vi "Moving Average (multiple).vi"(6 "Window Unit (points)":enum16{"Points", "Data"}(ring), 8 "error in (no error)":errorcluster, 10 "Window":dbl, 11 "XY-data":cluster{"X-array":dbl[], "Y-array":dbl[]}[](array[cluster])) -> (0 "error out":errorcluster, 3 "XY-data out":cluster{"X-array":dbl[], "Y-array":dbl[]}[](array[cluster]) {"Y-array" format="%.2p"; "X-array" format="%.2p"})   [LabVIEW 2019, in "xy_utilities.lvlib"]
doc: "Apply a moving average <b>XY-data</b>'s Y-Array according to <b>window</b>\n\nWire data to the data input to determine the polymorphic instance to use or manually select the instance."
uses:
  xy_utilities.lvlib
  Private/X Units.vi
  Private/X Array Range to Index.vi
  <vilib>/Analysis/3filter.llb/Smoothing Filter Coefficients.vi
  <vilib>/Analysis/3filter.llb/IIR Filter.vi
  <vilib>/Analysis/3filter.llb/IIR Filter (DBL).vi
  <vilib>/Utility/error.llb/Error Cluster From Error Code.vi
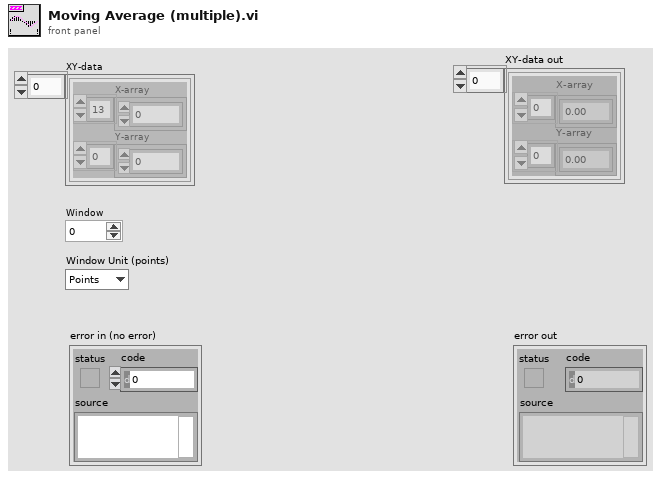
[diagram p1: front panel]
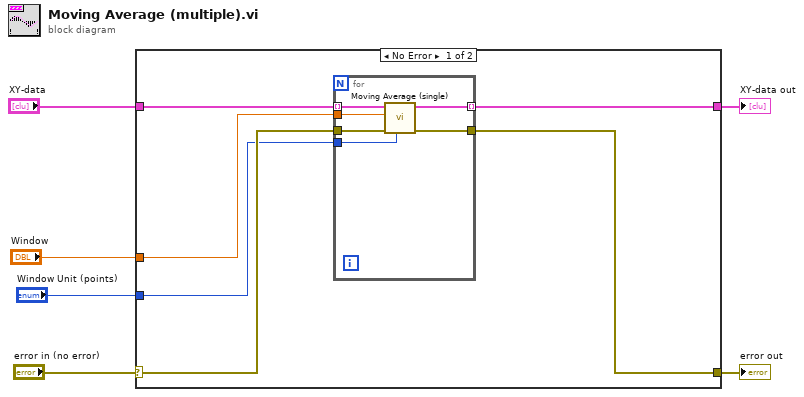
[diagram p0: block diagram]
diagram:
  n1 = case shown="No Error" "error in (no error)" {
    selector: "error in (no error)" -> [w9 w20]
    tunnel: [w8 w20] -> w5
    tunnel: "XY-data" -> [w12 w19]
    tunnel: [w11 w19] -> w3
    tunnel: "Window" -> [w10 _]
    tunnel: "Window Unit (points)" -> [w7 _]
    frame No Error {
      n2 = for {
        tunnel: w12 -> [w18] mode=indexing
        tunnel: [w17] -> w11 mode=indexing
        tunnel: w10 -> [w16]
        tunnel: w9 -> [w15]
        tunnel: [w14] -> w8
        tunnel: w7 -> [w13]
        n3 = call "Moving Average (single).vi"("Window Unit (points)"=w13, "error in (no error)"=w15, "Window"=w16, "XY-data"=w18) -> ("error out"=w14:errorcluster, "XY-data out"=w17:cluster{"X-array":dbl[], "Y-array":dbl[]})  [unwired: 6 in]
      }
    }
    frame Error {
    }
  }
  "error out" <- w5
  "XY-data out" <- w3
